vi "Set_Sub_Collection.vi"(8 "error in (no error)":errorcluster caption="entrée d'erreur (pas d'erreur)", 11 "Firebase PCBA en entrée":refnum<class "Firebase Benches.lvclass">) -> (0 "error out":errorcluster caption="sortie d'erreur", 3 "Firebase PCBA en sortie":refnum<class "Firebase Benches.lvclass">)   [LabVIEW 2020, in "Library Instrument & Equipement.lvlib" / "Library FireBase.lvlib" / "Firebase Benches.lvclass"]
doc: "Create New document\nPlease initialise the following values\n - Name BDD\n - Document of test sequence\n - API Key"
uses:
  Firebase Benches.lvclass
  C:/Users/ngarcin/OneDrive - Altyor/Standard TB/Class/Firebase/Source/Firebase Driver/Firebase Driver.lvclass
  Firebase Altyor/Firebase Altyor.lvclass
  Firebase Benches.lvclass/Firebase Benches.ctl
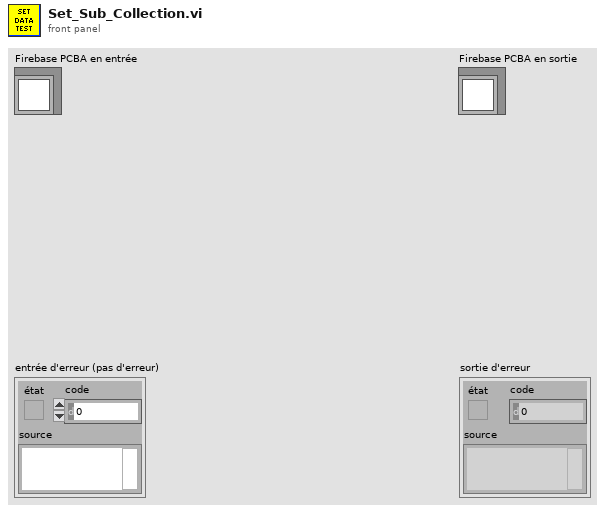
[diagram p1: front panel]
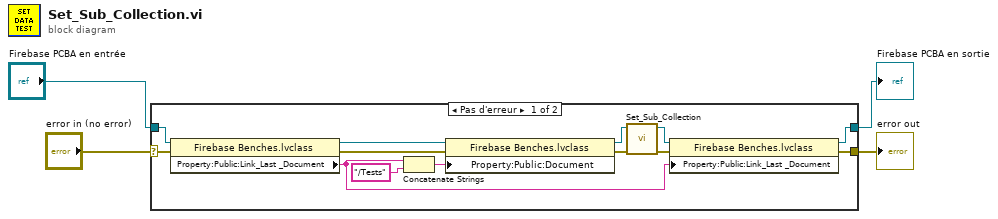
[diagram p0: block diagram]
diagram:
  n1 = case shown="Pas d'erreur" "error in (no error)" {
    selector: "error in (no error)" -> [w16 w19]
    tunnel: [w12 w19] -> w2
    tunnel: [w9 w18] -> w1
    tunnel: "Firebase PCBA en entrée" -> [w10 w18]
    frame No Error {
      n2 = property class="Firebase Benches.lvclass"(reference=w10, error in=w16) -> (reference out=w15:refnum<class "Firebase Benches.lvclass">, error out=w14:errorcluster, "Property:Public:Link_Last _Document"=w11:string)
      n3 = Concatenate Strings(w11, "/Tests" ("chaîne")) -> (w13:string)
      n4 = property class="Firebase Benches.lvclass"(reference=w15, error in=w14, "Property:Public:Document"=w13) -> (reference out=w5:refnum<class "Firebase Benches.lvclass">, error out=w8:errorcluster)
      n5 = call-parent "Set_Sub_Collection.vi"("error in (no error)"=w8, "Firebase PCBA en entrée"=w5) -> ("error out"=w7:errorcluster, "Firebase PCBA en sortie"=w6:refnum<class "Firebase Benches.lvclass">)  [unwired: 8 in]
      n6 = property class="Firebase Benches.lvclass"(reference=w6, error in=w7, "Property:Public:Link_Last _Document"=w11) -> (reference out=w9:refnum<class "Firebase Benches.lvclass">, error out=w12:errorcluster)
    }
    frame Error {
    }
  }
  "error out" <- w2
  "Firebase PCBA en sortie" <- w1
